vi "Clear Nodes.vi"(8 "error in (no error)":errorcluster, 11 "nodes":refnum<k20>[](array[refnum])) -> (0 "error out":errorcluster)   [LabVIEW 2017, in "Error File Management.lvlib"]
uses:
  Error File Management.lvlib
  <vilib>/xml/Close Reference(Node).vi
  <resource>/objmgr/DOMUserDefRef.rc
  <vilib>/xml/NI_XML.lvlib
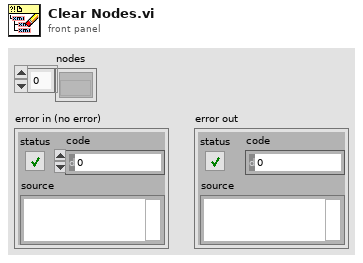
[diagram p1: front panel]
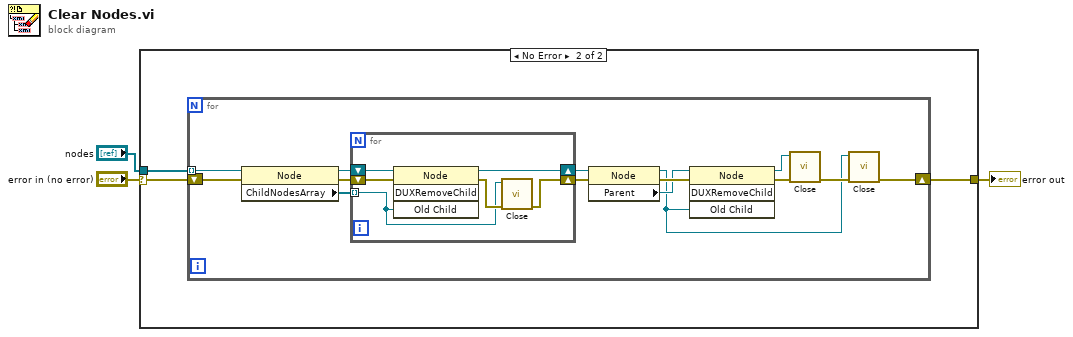
[diagram p0: block diagram]
diagram:
  n1 = case shown="No Error" "error in (no error)" {
    selector: "error in (no error)" -> [w4 w5]
    tunnel: "nodes" -> [_ w7]
    tunnel: [w4 w6] -> w1
    frame Error {
    }
    frame No Error {
      n2 = for {
        tunnel: w7 -> [w15] mode=indexing
        shift-right: [w8] -> w6
        shift-left: w5 -> [w14]
        n3 = property class="Node"(reference=w15, error in=w14) -> (reference out=w18:refnum<k20>, error out=w17:errorcluster, "ChildNodesArray"=w19:refnum<k20>[])
        n4 = for {
          tunnel: w19 -> [w23] mode=indexing
          shift-right: [w22] -> w13
          shift-left: w17 -> [w25]
          shift-right: [w24] -> w16
          shift-left: w18 -> [w26]
          n5 = invoke class="Node" method="DUXRemoveChild"(reference=w26, error in=w25, "Old Child"=w23) -> (reference out=w24:refnum<k20>, error out=w27:errorcluster)  [unwired: 1 in, 2 out]
          n6 = call-poly <vilib>:"Close.vi"("error in (no error)"=w27, "node"=w23) -> ("error out"=w22:errorcluster)  [unwired: 7 in]
        }
        n7 = property class="Node"(reference=w16, error in=w13) -> (reference out=w9:refnum<k20>, error out=w21:errorcluster, "Parent"=w20:refnum<k20>)
        n8 = invoke class="Node" method="DUXRemoveChild"(reference=w20, error in=w21, "Old Child"=w9) -> (reference out=w12:refnum<k20>, error out=w11:errorcluster)  [unwired: 1 in, 2 out]
        n9 = call-poly <vilib>:"Close.vi"("error in (no error)"=w11, "node"=w12) -> ("error out"=w10:errorcluster)  [unwired: 7 in]
        n10 = call-poly <vilib>:"Close.vi"("error in (no error)"=w10, "node"=w9) -> ("error out"=w8:errorcluster)  [unwired: 7 in]
      }
    }
  }
  "error out" <- w1
